vi "Hide Panel.vi"(8 "error in (no error)":errorcluster) -> (0 "error out":errorcluster)   [LabVIEW 2015, in "Collect Data Mgr.lvlib"]
doc: "Send the Hide Panel request to the Module's Main.vi.\n_____\nBased on Delacor QMH Project Template 2.1.0.2."
uses:
  Collect Data Mgr.lvlib
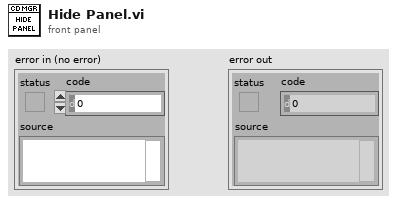
[diagram p1: front panel]
types:
  T1 = typedef "Collect Data Mgr.lvlib/Request Events--cluster.ctl" = cluster{"Stop Module":refnum<user-event>, "Show Panel":refnum<user-event>, "Hide Panel":refnum<user-event>, "Get Module Execution Status":refnum<user-event>, "Show Diagram":refnum<user-event>, "Start Collect":refnum<user-event>, "Stop Collect":refnum<user-event>}
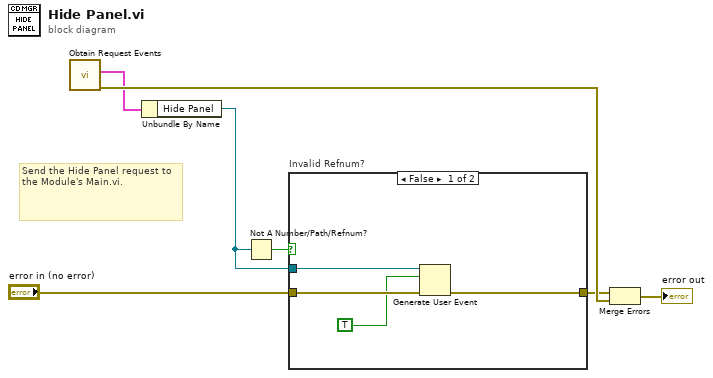
[diagram p0: block diagram]
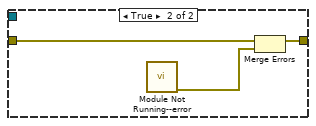
[diagram p2: hidden frame]
diagram:
  # "Send the Hide Panel request to the Module's Main.vi."
  n1 = call "Obtain Request Events.vi"() -> ("error out"=w6:errorcluster, "Probe Mgr Request Events"=w5:T1)  [unwired: 10 in]
  n2 = Unbundle By Name(w5) -> ("Hide Panel"=w3:refnum<user-event>)
  n3 = Not A Number/Path/Refnum?(number/path/refnum=w3) -> (NaN/Path/Refnum?=w4:bool)
  n4 = case "Invalid Refnum?" shown="False" w4 {
    tunnel: "error in (no error)" -> [w11 w12]
    tunnel: [w10 w13] -> w1
    tunnel: w3 -> [w9 _]
    frame False {
      n5 = Generate User Event(user event=w9, event data cluster=TRUE ("event data"), error in=w11) -> (error out=w10:errorcluster)  [unwired: 1 in, 1 out]
    }
    frame True {
      n6 = call "Module Not Running--error.vi"() -> ("error out"=w14:errorcluster)  [unwired: 11 in]
      n7 = Merge Errors(w12, w14) -> (w13:errorcluster)
    }
  }
  n8 = Merge Errors(w1, w6) -> (→"error out":errorcluster)
